vi "sv_Buffer XY Data (M by N).vi"(0 "XY signals":cluster{"X":dbl[], "Y":dbl[]}[][](array[cluster]) {"X" format="%.2f"; "Y" format="%.2f"}, 2 "reset? (F)":bool, 11 "error in (no error)":errorcluster, 12 "buffer settings":T1 {"buffer mode" items=["Infinite length", "Last block data", "Custom"]}) -> (4 "buffered XY signals":cluster{"X":dbl[], "Y":dbl[]}[][](array[cluster]) {"X" format="%.2f"; "Y" format="%.2f"}, 15 "error out":errorcluster)   [LabVIEW 2017]
doc: "Buffers the input signals and returns them in first-in first-out (FIFO) mode. The data type you wire to the <B>XY signal</B> input determines the polymorphic instance to use."
uses:
  <vilib>/addons/_NISVFA/_Shared subVIs/Controls/sv_Buffer XY Settings.ctl
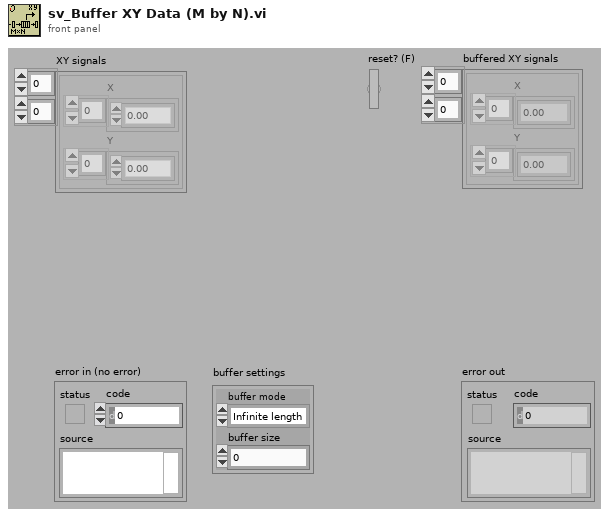
[diagram p1: front panel]
types:
  T1 = typedef "sv_Buffer XY Settings.ctl" = cluster{"buffer mode":u16, "buffer size":dbl}
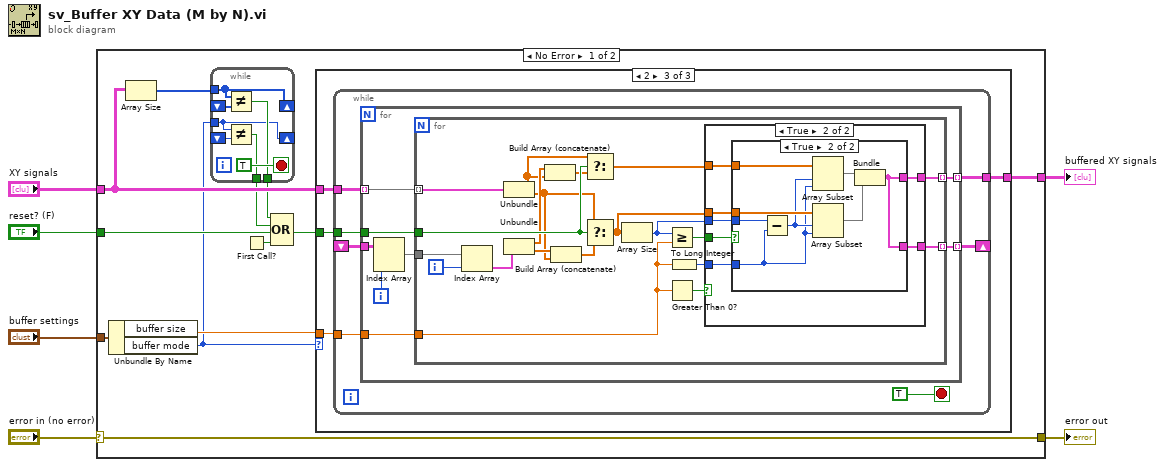
[diagram p0: block diagram]
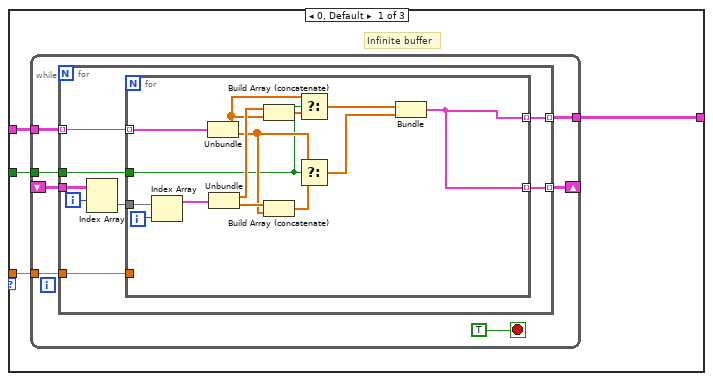
[diagram p2: hidden frame]
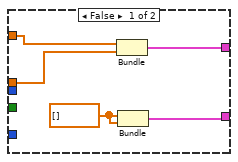
[diagram p4: hidden frame]
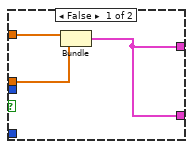
[diagram p5: hidden frame]
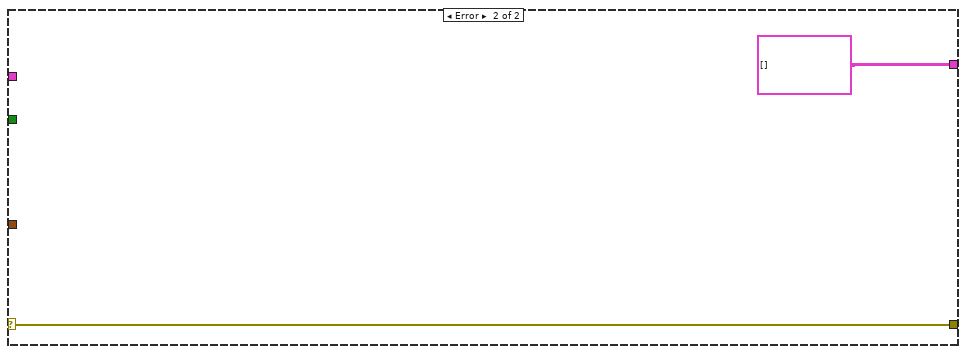
[diagram p6: hidden frame]
diagram:
  n1 = case shown="No Error" "error in (no error)" {
    selector: "error in (no error)" -> [w11 w123]
    tunnel: [w11 w123] -> w4
    tunnel: "buffer settings" -> [w18 _]
    tunnel: "XY signals" -> [w16 _]
    tunnel: "reset? (F)" -> [w14 _]
    tunnel: [w17 cluster{"X":dbl[], "Y":dbl[]}[][] []] -> w3
    frame No Error {
      n2 = Unbundle By Name(w18) -> ("buffer size"=w10:dbl, "buffer mode"=w9:u16)
      n3 = Array Size(array=w16) -> (size(s)=w15:i32[])
      n4 = while {
        tunnel: w15 -> [w25]
        shift-right: [w25] -> _
        shift-left: _ -> [w22]
        tunnel: [w23] -> w8
        shift-right: [w21] -> _
        shift-left: _ -> [w20]
        tunnel: w9 -> [w21]
        tunnel: [w19] -> w7
        stop <- TRUE stop-if-true
        n5 = Not Equal?(x=w25, y=w22) -> (x != y?=w23:bool)
        n6 = Not Equal?(x=w21, y=w20) -> (x != y?=w19:bool)
      }
      n7 = First Call?() -> (First Call?: T/F=w13:bool)
      n8 = Compound Arithmetic op=OR(w8, w7, w14, w13) -> (w12:bool)
      n9 = case shown="2" w9 {
        tunnel: w10 -> [w29 _ w61]
        tunnel: w16 -> [w27 w59 w63]
        tunnel: w12 -> [w26 _ w62]
        tunnel: [w28 w59 w60] -> w17
        frame 0, Default {
          # "Infinite buffer"
          n10 = while {
            tunnel: w29 -> [w33]
            tunnel: [w36] -> w28
            tunnel: w27 -> [w31]
            shift-right: [w35] -> _
            shift-left: _ -> [w32]
            tunnel: w26 -> [w30]
            stop <- TRUE stop-if-true
            n11 = for {
              tunnel: [w44] -> w36 mode=indexing
              tunnel: [w37] -> w35 mode=indexing
              tunnel: w33 -> [w38]
              tunnel: w32 -> [w42]
              tunnel: w31 -> [w43] mode=indexing
              tunnel: w30 -> [w39]
              i -> [w40]
              n12 = Index Array(array=w42, index (row)=w40) -> (element=w41:cluster{"X":dbl[], "Y":dbl[]}[])  [unwired: 1 in]
              n13 = for {
                tunnel: [w45] -> w44 mode=indexing
                tunnel: w43 -> [w52] mode=indexing
                tunnel: w41 -> [w50]
                tunnel: w39 -> [w49]
                tunnel: w38 -> [_]
                tunnel: [w45] -> w37 mode=indexing
                i -> [w46]
                n14 = Index Array(array=w50, index=w46) -> (element=w47:cluster{"X":dbl[], "Y":dbl[]})
                n15 = Unbundle(w52) -> ("X"=w57:dbl[], "Y"=w54:dbl[])
                n16 = Unbundle(w47) -> ("X"=w58:dbl[], "Y"=w55:dbl[])
                n17 = Build Array (concatenate)(w58, w57) -> (w56:dbl[])
                n18 = Build Array (concatenate)(w55, w54) -> (w53:dbl[])
                n19 = Select(t=w57, s=w49, f=w56) -> (s? t:f=w48:dbl[])
                n20 = Select(t=w54, s=w49, f=w53) -> (s? t:f=w51:dbl[])
                n21 = Bundle("X"=w48, "Y"=w51) -> (w45:cluster{"X":dbl[], "Y":dbl[]})  [unwired: 1 in]
              }
            }
          }
        }
        frame 1 {
          # "Last block"
        }
        frame 2 {
          n22 = while {
            tunnel: w63 -> [w70]
            shift-right: [w66] -> _
            shift-left: _ -> [w64]
            tunnel: w62 -> [w67]
            tunnel: w61 -> [w68]
            tunnel: [w65] -> w60
            stop <- TRUE stop-if-true
            n23 = for {
              tunnel: w70 -> [w78] mode=indexing
              tunnel: w68 -> [w71]
              tunnel: w67 -> [w77]
              tunnel: [w76] -> w66 mode=indexing
              tunnel: [w75] -> w65 mode=indexing
              tunnel: w64 -> [w74]
              i -> [w73]
              n24 = Index Array(array=w74, index (row)=w73) -> (element=w72:cluster{"X":dbl[], "Y":dbl[]}[])  [unwired: 1 in]
              n25 = for {
                tunnel: w78 -> [w98] mode=indexing
                tunnel: w77 -> [w94]
                tunnel: [w92] -> w76 mode=indexing
                tunnel: [w91] -> w75 mode=indexing
                tunnel: w72 -> [w83]
                tunnel: w71 -> [w81]
                i -> [w79]
                n26 = Index Array(array=w83, index=w79) -> (element=w80:cluster{"X":dbl[], "Y":dbl[]})
                n27 = Unbundle(w98) -> ("X"=w88:dbl[], "Y"=w85:dbl[])
                n28 = Unbundle(w80) -> ("X"=w89:dbl[], "Y"=w86:dbl[])
                n29 = Build Array (concatenate)(w89, w88) -> (w87:dbl[])
                n30 = Build Array (concatenate)(w86, w85) -> (w84:dbl[])
                n31 = Select(t=w88, s=w94, f=w87) -> (s? t:f=w93:dbl[])
                n32 = Select(t=w85, s=w94, f=w84) -> (s? t:f=w97:dbl[])
                n33 = Array Size(array=w97) -> (size(s)=w96:i32)
                n34 = Greater Or Equal?(x=w96, y=w81) -> (x >= y?=w90:bool)
                n35 = Greater Than 0?(x=w81) -> (x > 0?=w82:bool)
                n36 = To Long Integer(number=w81) -> (32bit integer=w95:i32)
                n37 = case shown="True" w82 {
                  tunnel: w97 -> [w102 w110]
                  tunnel: w96 -> [_ w109]
                  tunnel: w95 -> [_ w108]
                  tunnel: w93 -> [w103 w107]
                  tunnel: [w99 w106] -> w92
                  tunnel: [w101 w105] -> w91
                  tunnel: w90 -> [_ w104]
                  frame False {
                    w100 = dbl[] [] ("Y")
                    n38 = Bundle("X"=w103, "Y"=w102) -> (w101:cluster{"X":dbl[], "Y":dbl[]})  [unwired: 1 in]
                    n39 = Bundle("Y"=w100, "Y"=w100) -> (w99:cluster{"Y":dbl[], "Y":dbl[]})  [unwired: 1 in]
                  }
                  frame True {
                    n40 = case shown="True" w104 {
                      tunnel: w110 -> [w112 w121]
                      tunnel: w108 -> [_ w117]
                      tunnel: w109 -> [_ w120]
                      tunnel: w107 -> [w113 w119]
                      tunnel: [w111 w114] -> w106
                      tunnel: [w111 w114] -> w105
                      frame False {
                        n41 = Bundle("X"=w113, "Y"=w112) -> (w111:cluster{"X":dbl[], "Y":dbl[]})  [unwired: 1 in]
                      }
                      frame True {
                        n42 = Subtract(x=w120, y=w117) -> (x-y=w118:i32)
                        n43 = Array Subset(array=w119, index=w118, length=w117) -> (w116:dbl[])
                        n44 = Array Subset(array=w121, index=w118, length=w117) -> (w115:dbl[])
                        n45 = Bundle(w116, w115) -> (w114:cluster{dbl[], dbl[]})  [unwired: 1 in]
                      }
                    }
                  }
                }
              }
            }
          }
        }
      }
    }
    frame Error {
    }
  }
  "error out" <- w4
  "buffered XY signals" <- w3
